vi "ni579x Verify Compatibility.vi"(0 "Register Bus":T1, 11 "Error In":errorcluster) -> (4 "Register Bus (out)":T1, 15 "Error Out":errorcluster)   [LabVIEW 2015, in "ni579x Config v2 Host.lvlib"]
uses:
  <instrlib>/ni579x/Config/v2/Host/ni579x Config v2 Host.lvlib
  <instrlib>/_niInstr/Register Bus/v0/Host/Public/Register Bus Session.ctl
  <instrlib>/_niInstr/Register Bus/v0/Host/Private/Session Data.ctl
  <instrlib>/ni579x/Config/v2/Shared/Types/ni579x User Command.ctl
  <instrlib>/ni579x/Config/v2/Shared/Types/ni579x User Command ID.ctl
  <instrlib>/_niInstr/Register Bus/v0/Host/Public/Register Read Request.ctl
  <instrlib>/ni579x/Config/v2/Shared/Types/ni579x Register Bus Subsystem ID.ctl
  <instrlib>/ni579x/Config/v2/Shared/ni579x Config v2 Shared.lvlib
  <instrlib>/_niInstr/Register Bus/v0/Host/niInstr Register Bus v0 Host.lvlib
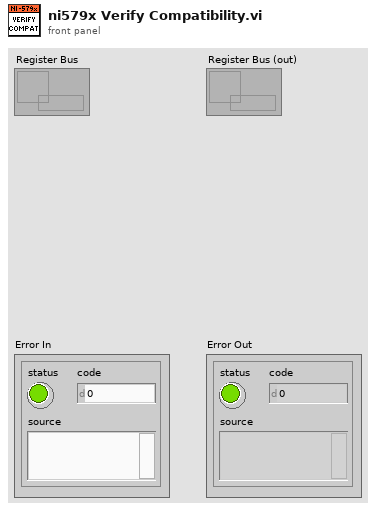
[diagram p1: front panel]
types:
  T1 = typedef "niInstr Register Bus v0 Host.lvlib/Register Bus Session.ctl" = refnum<queue>
  T2 = typedef "niInstr Register Bus v0 Host.lvlib/Register Read Request.ctl" = cluster{"subsystem":u8, "address":u16}
  T3 = typedef "ni579x Config v2 Shared.lvlib/ni579x User Command.ctl" = cluster{"User Data 0":u8, "User Data 1":u8, "User Command ID":T4}
  T4 = typedef "ni579x Config v2 Shared.lvlib/ni579x User Command ID.ctl" = u8
  T5 = typedef "ni579x Config v2 Shared.lvlib/ni579x Register Bus Subsystem ID.ctl" = u8
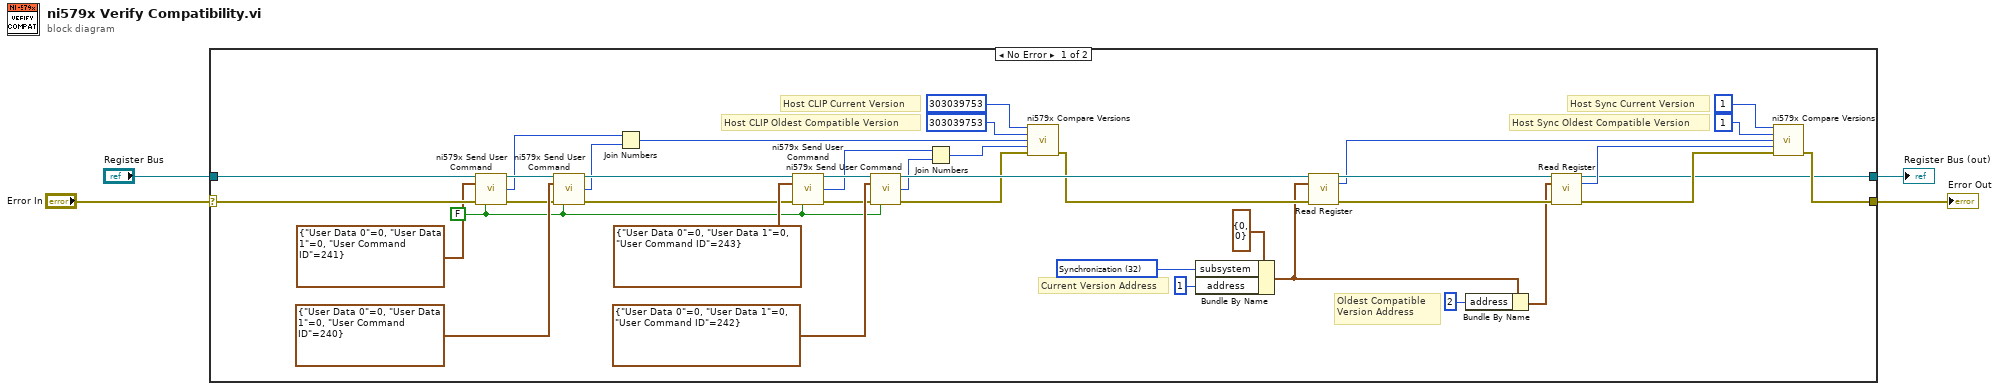
[diagram p0: block diagram]
diagram:
  n1 = case shown="No Error" "Error In" {
    selector: "Error In" -> [w42 w45]
    tunnel: [w22 w45] -> w3
    tunnel: "Register Bus" -> [w43 w44]
    tunnel: [w21 w44] -> w1
    frame No Error {
      w7 = FALSE ("wait for completion?")
      w35 = T5 32 items=["FAM Register Operation"=0, "User Command"=16, "Synchronization"=32] ("Subsystem ID")
      # "Host CLIP Oldest Compatible Version"
      # "Host CLIP Current Version"
      # "Host Sync Oldest Compatible Version"
      # "Host Sync Current Version"
      # "Oldest Compatible \nVersion Address"
      # "Current Version Address"
      n2 = call <instrlib>:"ni579x Send User Command.vi"("Register Bus"=w43, "User Command"=T3 {"User Data 0"=0, "User Data 1"=0, "User Command ID"=241}, "Error In"=w42, "wait for completion?"=w7) -> ("Register Bus (out)"=w20:T1, "user return value"=w14:u16, "Error Out"=w19:errorcluster)  [unwired: 7 in, 2 out]
      n3 = call <instrlib>:"ni579x Send User Command.vi"("Register Bus"=w20, "User Command"=T3 {"User Data 0"=0, "User Data 1"=0, "User Command ID"=240}, "Error In"=w19, "wait for completion?"=w7) -> ("Register Bus (out)"=w16:T1, "user return value"=w13:u16, "Error Out"=w15:errorcluster)  [unwired: 7 in, 2 out]
      n4 = Join Numbers(hi=w14, lo=w13) -> ((hi.lo)=w10:u32)
      n5 = call <instrlib>:"ni579x Send User Command.vi"("Register Bus"=w16, "User Command"=T3 {"User Data 0"=0, "User Data 1"=0, "User Command ID"=243}, "Error In"=w15, "wait for completion?"=w7) -> ("Register Bus (out)"=w17:T1, "user return value"=w12:u16, "Error Out"=w18:errorcluster)  [unwired: 7 in, 2 out]
      n6 = call <instrlib>:"ni579x Send User Command.vi"("Register Bus"=w17, "User Command"=T3 {"User Data 0"=0, "User Data 1"=0, "User Command ID"=242}, "Error In"=w18, "wait for completion?"=w7) -> ("Register Bus (out)"=w37:T1, "user return value"=w11:u16, "Error Out"=w8:errorcluster)  [unwired: 7 in, 2 out]
      n7 = Join Numbers(hi=w12, lo=w11) -> ((hi.lo)=w9:u32)
      n8 = call <instrlib>:"ni579x Compare Versions.vi"("Host Current Version"=u32 303039753, "Host Oldest Compatible Version"=u32 303039753 ("Host Current Version"), "FPGA Current Version"=w10, "FPGA Oldest Compatible Version"=w9, "Error In"=w8) -> ("Error Out"=w36:errorcluster)  [unwired: 10 in]
      n9 = Bundle By Name(cluster=T2 {"subsystem"=0, "address"=0} ("register read request"), "subsystem"=w35, "address"=u16 1) -> (w30:T2)
      n10 = call <instrlib>:"Read Register.vi"("session in"=w37, "register read request"=w30, "error in"=w36) -> ("session out"=w32:T1, "data"=w24:u32, "error out"=w31:errorcluster)  [unwired: 10 in]
      n11 = Bundle By Name(cluster=w30, "address"=u16 2) -> (w28:T2)
      n12 = call <instrlib>:"Read Register.vi"("session in"=w32, "register read request"=w28, "error in"=w31) -> ("session out"=w21:T1, "data"=w23:u32, "error out"=w25:errorcluster)  [unwired: 10 in]
      n13 = call <instrlib>:"ni579x Compare Versions.vi"("Host Current Version"=u32 1, "Host Oldest Compatible Version"=u32 1 ("Host Current Version"), "FPGA Current Version"=w24, "FPGA Oldest Compatible Version"=w23, "Error In"=w25) -> ("Error Out"=w22:errorcluster)  [unwired: 10 in]
    }
    frame Error {
    }
  }
  "Register Bus (out)" <- w1
  "Error Out" <- w3
